vi "Measurement_nm.vi"() -> ()   [LabVIEW 2011]
uses:
  <userlib>/LV-LINK/PolySubVIs/CreateAinChan.vi
  <userlib>/LV-LINK/PolySubVIs/OLTimingSetInput.vi
  <userlib>/LV-LINK/PolySubVIs/OLReadMultiple2D.vi
  <userlib>/LV-LINK/PolySubVIs/OLTriggerDigital.vi
panel:
  out "error out 4":errorcluster
  out "error out 2":errorcluster
  out "error out 3":errorcluster
  out "Acquired Data 2":dbl[][](graph)=[[-5.8099365234375, -4.9749755859375, -3.653564453125, -1.9744873046875, -0.10223388671875, 1.7791748046875, 3.48602294921875, 4.85198974609375, 5.74188232421875, 6.07025146484375, 5.80322265625, 4.97039794921875, 3.6492919921875, 1.9720458984375, 0.0982666015625, -1.78375244140625, -3.49151611328125, -4.8583984375, -5.74920654296875, -6.077880859375, -5.81329345703125, -4.97955322265625, -3.6572265625, -1.97845458984375, -0.1068115234375, 1.77398681640625, 3.48297119140625, 4.8492431640625, 5.7403564453125, 6.06903076171875, 5.80474853515625, 4.97283935546875, 3.6529541015625, 1.9757080078125, 0.10345458984375, -1.778564453125, -3.48876953125, -4.85443115234375, -5.74737548828125, -6.07757568359375, -5.81390380859375, -4.9810791015625, -3.66180419921875, -1.983642578125, -0.11077880859375, 1.77093505859375, 3.47747802734375, 4.8455810546875, 5.73974609375, 6.0699462890625, 5.80718994140625, 4.97528076171875, 3.65631103515625, 1.97967529296875, 0.10772705078125, -1.77398681640625, -3.48236083984375, -4.85137939453125, -5.7452392578125, -6.07666015625, -5.81451416015625, -4.98443603515625, -3.66546630859375, -1.98760986328125, -0.11688232421875, 1.76513671875, 3.47442626953125, 4.84283447265625, 5.73760986328125, 6.06964111328125, 5.80780029296875, 4.97772216796875, 3.65966796875, 1.9842529296875, 0.11199951171875, -1.76910400390625, -3.48052978515625, -4.84771728515625, -5.74462890625, -6.07818603515625, -5.8154296875, -4.9871826171875, -3.6688232421875, -1.99249267578125, -0.12115478515625, 1.76055908203125, 3.47198486328125, 4.84039306640625, 5.736083984375, 6.07025146484375, 5.8074951171875, 4.9798583984375, 3.66424560546875, 1.98760986328125, 0.1190185546875, -1.76513671875, -3.47625732421875, -4.8455810546875, -5.7440185546875, -6.07818603515625]] caption="Acquired Data"
  out "Sample Freq":dbl=40000.0
  in  "Number of cycles":dbl=5.0
  out "Actual Sample Freq":dbl=40000.0
  in  "Samples per cycle":dbl=20.0
  in  "Vin Max":dbl=10.0
  in  "Vin Min":dbl=-10.0
  in  "Device Name":refnum<visa-resource-name>="USB0::0x0699::0x0347::C036837::INSTR"
  in  "error in":errorcluster
  out "error out":errorcluster
  out "VISA resource name out":refnum<visa-resource-name>="USB0::0x0699::0x0347::C036837::INSTR"
  in  "Jet Freq":dbl=2000.0
  in  "Amplitude Delta":dbl=1.0
  in  "Min Amplitude":dbl=3.0
  in  "Max Amplitude":dbl=6.0
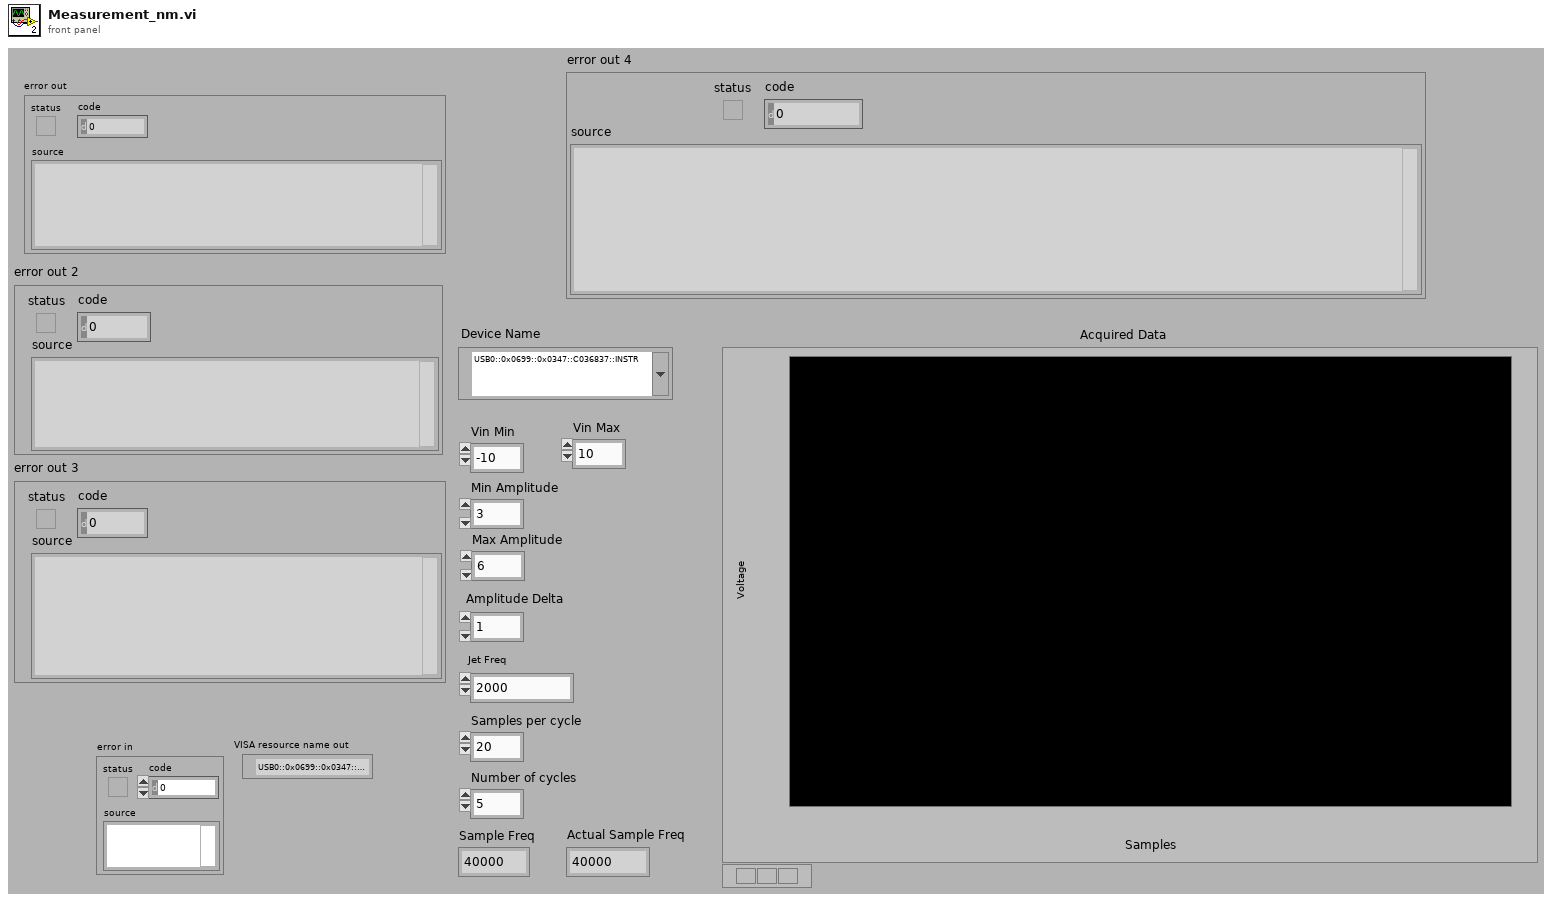
[diagram p1: front panel]
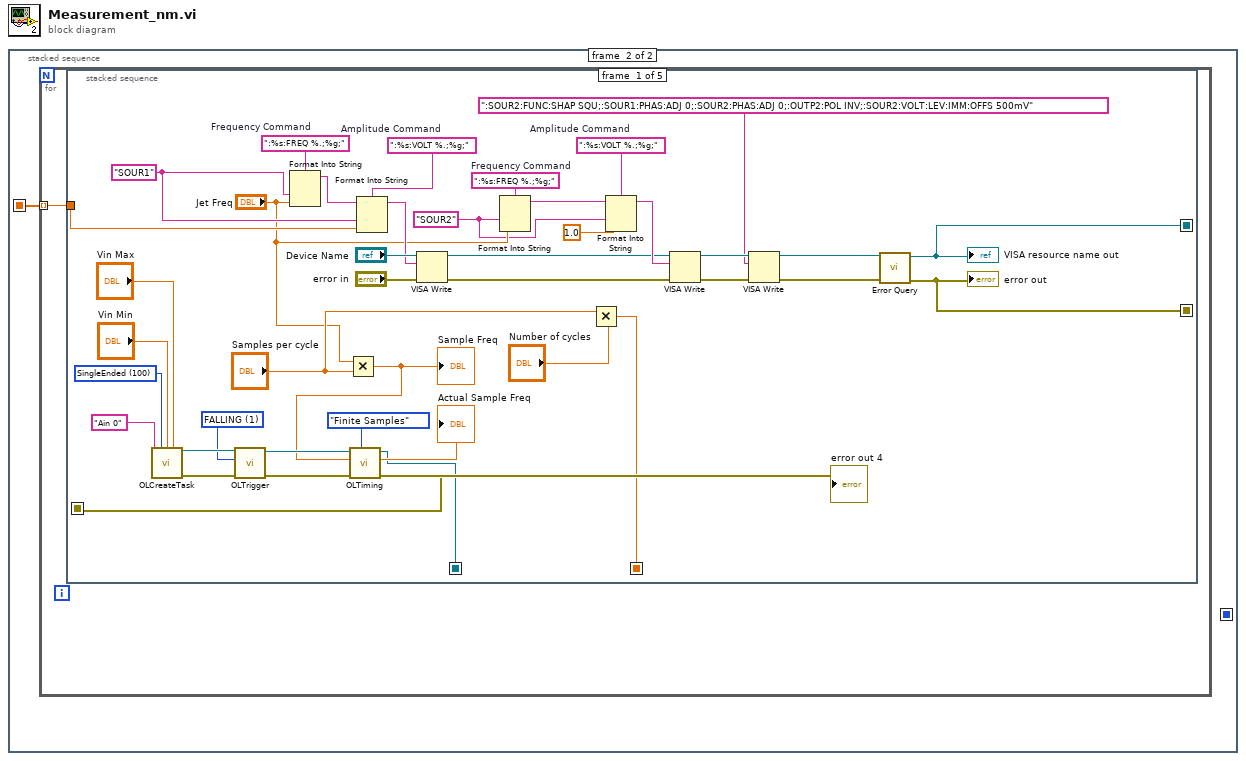
[diagram p0: block diagram]
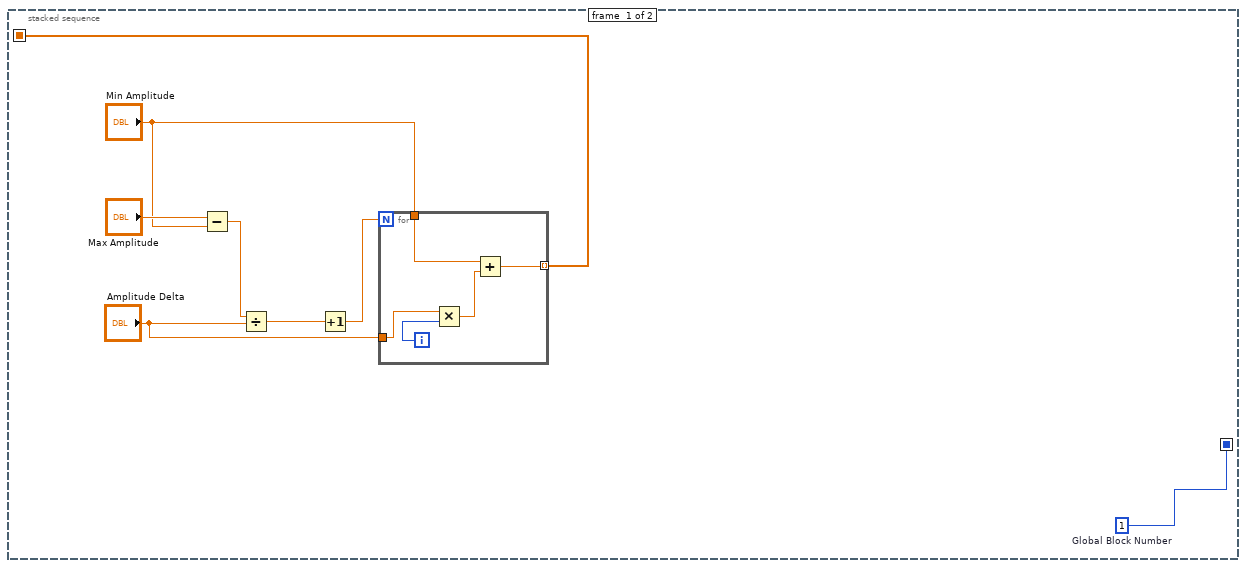
[diagram p2: hidden frame]
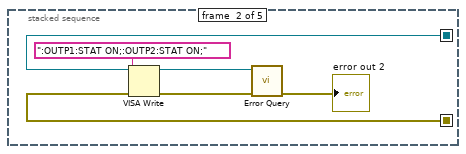
[diagram p3: hidden frame]
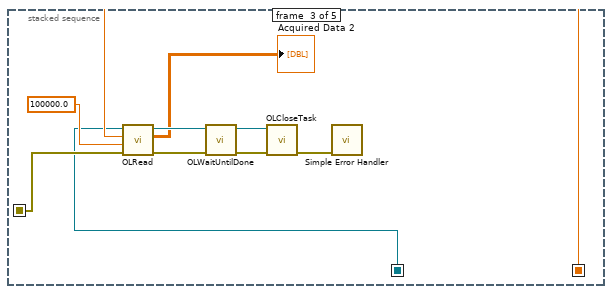
[diagram p4: hidden frame]
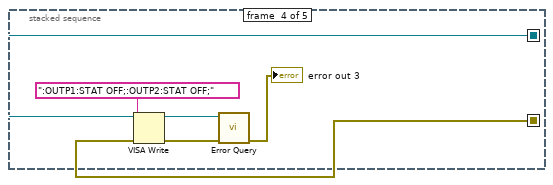
[diagram p5: hidden frame]
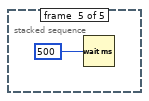
[diagram p6: hidden frame]
diagram:
  n1 = stacked-sequence {
    seq-local: [w2 _] -> [_ w14]
    seq-local: [w1 _] -> [_ _]
    frame #0 {
      w1 = 1  # Global Block Number
      n2 = Subtract(x="Max Amplitude", y="Min Amplitude") -> (x-y=w8:dbl)
      n3 = Divide(x=w8, y="Amplitude Delta") -> (x/y=w6:dbl)
      n4 = Increment(x=w6) -> (x+1=w5:dbl)
      n5 = for {
        N: w5 -> [_]
        tunnel: [w12] -> w2 mode=indexing
        tunnel: "Min Amplitude" -> [w9]
        tunnel: "Amplitude Delta" -> [w11]
        i -> [w13]
        n6 = Multiply(x=w11, y=w13) -> (x*y=w10:dbl)
        n7 = Add(x=w9, y=w10) -> (x+y=w12:dbl)
      }
    }
    frame #1 {
      n8 = for {
        tunnel: w14 -> [w15] mode=indexing
        n9 = stacked-sequence {
          seq-local: [w24 _ _ _ _] -> [_ _ w65 _ _]
          seq-local: [w23 _ _ _ _] -> [_ _ w63 _ _]
          seq-local: [w22 _ _ _ _] -> [_ _ w64 _ _]
          seq-local: [w20 _ _ _ _] -> [_ w59 _ w74 _]
          seq-local: [w21 _ _ _ _] -> [_ w58 _ w73 _]
          tunnel: w15 -> [w55 _ _ _ _]
          frame #0 {
            w17 = "SOUR2" ("input 1")
            w19 = ":%s:FREQ %.;%g;"  # Frequency Command
            w31 = 1 items=["RISING", "FALLING"] ("External Trigger Polarity")
            w38 = 100 items=["SingleEnded"=100, "Differential"=101] ("Channel Type")
            w47 = ":%s:VOLT %.;%g;"  # Amplitude Command
            w54 = ":%s:FREQ %.;%g;"  # Frequency Command
            w53 = "SOUR1" ("input 1")
            w56 = ":%s:VOLT %.;%g;"  # Amplitude Command
            n10 = call-poly <userlib>:"OLCreateTask.vi"("Channel Type"=w38, "Range Min"="Vin Min", "Range Max"="Vin Max", "Channel"="Ain 0") -> ("Task Out"=w33:refnum<k24>, "error out"=w32:errorcluster)  [unwired: 10 in]
            "error out 4" <- w32
            n11 = call-poly <userlib>:"OLTrigger.vi"("error in (no error)"=w32, "External Trigger Polarity"=w31, "Task In"=w33) -> ("error out"=w30:errorcluster, "Task Out"=w29:refnum<k24>)  [unwired: 7 in]
            n12 = Format Into String(format string=w54, w53, "Jet Freq") -> (resulting string=w49:string)  [unwired: 2 in, 1 out]
            n13 = Multiply(x="Jet Freq", y="Samples per cycle") -> (x*y=w27:dbl)
            "Sample Freq" <- w27
            n14 = call-poly <userlib>:"OLTiming.vi"("Sample Mode"=enum16{"Finite Samples", "Continuous Samples"}."Finite Samples", "error in (no error)"=w30, "Sample Freq (Hz)"=w27, "Task In"=w29) -> ("error out"=w22:errorcluster, "Actual Sample Freq"=→"Actual Sample Freq":dbl, "Task Out"=w23:refnum<k24>)  [unwired: 5 in]
            n15 = Format Into String(format string=w56, initial string=w49, w53, w55) -> (resulting string=w50:string)  [unwired: 1 in, 1 out]
            n16 = VISA Write(VISA resource name="Device Name", write buffer=w50, error in (no error)="error in") -> (VISA resource name out=w44:refnum<visa-resource-name>, error out=w45:errorcluster)  [unwired: 1 out]
            n17 = Format Into String(format string=w19, w17, "Jet Freq") -> (resulting string=w16:string)  [unwired: 2 in, 1 out]
            n18 = Multiply(x="Samples per cycle", y="Number of cycles") -> (x*y=w24:dbl)
            n19 = Format Into String(format string=w47, initial string=w16, w17, 1.0 ("input 2")) -> (resulting string=w48:string)  [unwired: 1 in, 1 out]
            n20 = VISA Write(VISA resource name=w44, write buffer=w48, error in (no error)=w45) -> (VISA resource name out=w43:refnum<visa-resource-name>, error out=w41:errorcluster)  [unwired: 1 out]
            n21 = VISA Write(VISA resource name=w43, write buffer=":SOUR2:FUNC:SHAP SQU;:SOUR1:PHAS:ADJ 0;:SOUR2:PHAS:ADJ 0;:OUTP2:POL INV;:SOUR2:VOLT:LEV:IMM:OFFS 500mV", error in (no error)=w41) -> (VISA resource name out=w42:refnum<visa-resource-name>, error out=w40:errorcluster)  [unwired: 1 out]
            n22 = call <instrlib>:"Error Query.vi"("error in (no error)"=w40, "VISA resource name"=w42) -> ("error out"=w21:errorcluster, "VISA resource name out"=w20:refnum<visa-resource-name>)  [unwired: 6 in, 2 out]
            "error out" <- w21
            "VISA resource name out" <- w20
          }
          frame #1 {
            n23 = VISA Write(VISA resource name=w59, write buffer=":OUTP1:STAT ON;:OUTP2:STAT ON;", error in (no error)=w58) -> (VISA resource name out=w61:refnum<visa-resource-name>, error out=w62:errorcluster)  [unwired: 1 out]
            n24 = call <instrlib>:"Error Query.vi"("error in (no error)"=w62, "VISA resource name"=w61) -> ("error out"=→"error out 2":errorcluster)  [unwired: 6 in, 3 out]
          }
          frame #2 {
            n25 = call-poly <userlib>:"OLRead.vi"("error in (no error)"=w64, "Timeout"=100000.0, "Samples Per Channel"=w65, "Task In"=w63) -> ("error out"=w67:errorcluster, "ReadData"=→"Acquired Data 2":dbl[][], "Task Out"=w68:refnum<k24>)  [unwired: 5 in]
            n26 = call <userlib>:"OLWaitUntilDone.vi"("error in"=w67, "Task In"=w68) -> ("error out"=w70:errorcluster, "Task Out"=w69:refnum<k24>)  [unwired: 8 in]
            n27 = call <userlib>:"OLCloseTask.vi"("Error in"=w70, "Task In"=w69) -> ("Error Out"=w71:errorcluster)  [unwired: 9 in]
            n28 = call <vilib>:"Simple Error Handler.vi"("error in (no error)"=w71) -> ()  [unwired: 4 in, 5 out]
          }
          frame #3 {
            n29 = VISA Write(VISA resource name=w74, write buffer=":OUTP1:STAT OFF;:OUTP2:STAT OFF;", error in (no error)=w73) -> (VISA resource name out=w76:refnum<visa-resource-name>, error out=w75:errorcluster)  [unwired: 1 out]
            n30 = call <instrlib>:"Error Query.vi"("error in (no error)"=w75, "VISA resource name"=w76) -> ("error out"=→"error out 3":errorcluster)  [unwired: 6 in, 3 out]
          }
          frame #4 {
            n31 = Wait (ms)(milliseconds to wait=u32 500) -> ()  [unwired: 1 out]
          }
        }
      }
    }
  }
